vi "RampStateMachine.vi"(8 "error in (no error)":errorcluster) -> (0 "error out":errorcluster)   [LabVIEW 2013]
doc: "Use this template to build a VI to use as a subVI."
uses:
  RampProgramModel/RampProgramModel.lvclass
  RampState.ctl
  RampProgramModel/RampProgramModel.lvclass/RampProgramModel.ctl
  <vilib>/Utility/file.llb/Read From Spreadsheet File (DBL).vi
  <vilib>/Utility/file.llb/Write To Spreadsheet File (string).vi
panel:
  in  "Clear Table":bool
  in  "Repeat Program":u32=1 min=1 max=1000 step=1
  out "Current Repeat":u32=1 min=1 max=1000 step=1
  out "Repeat Program ind":u32=1 min=1 max=1000 step=1
  in  "SaveProgram":bool
  in  "LoadProgram":bool
  in  "PauseProgram":bool
  out "Time Elapsed":dbl
  out "Cooling rate (°C/min)":dbl
  out "SP (°C)":dbl
  in  "StopProgram":bool
  in  "RunProgram":bool
  in  "Current Temperature":dbl(slide) scale=-50.0..20.0 scale format="%.1g"
  out "Status":string
  in  "stop":bool
  in  "Add Entry":bool
  out "Ramp Program Table":string[][](table)
  # "Hardware Abstraction"
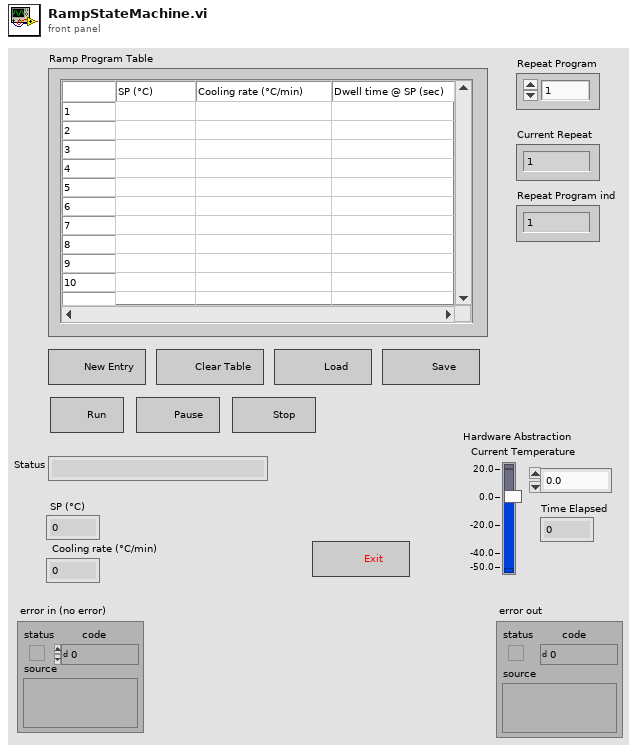
[diagram p1: front panel]
types:
  T1 = typedef "RampState.ctl" = enum16{"Pause Program", "Heatling/Cooling", "Dwelling @ SP", "Stopped"}
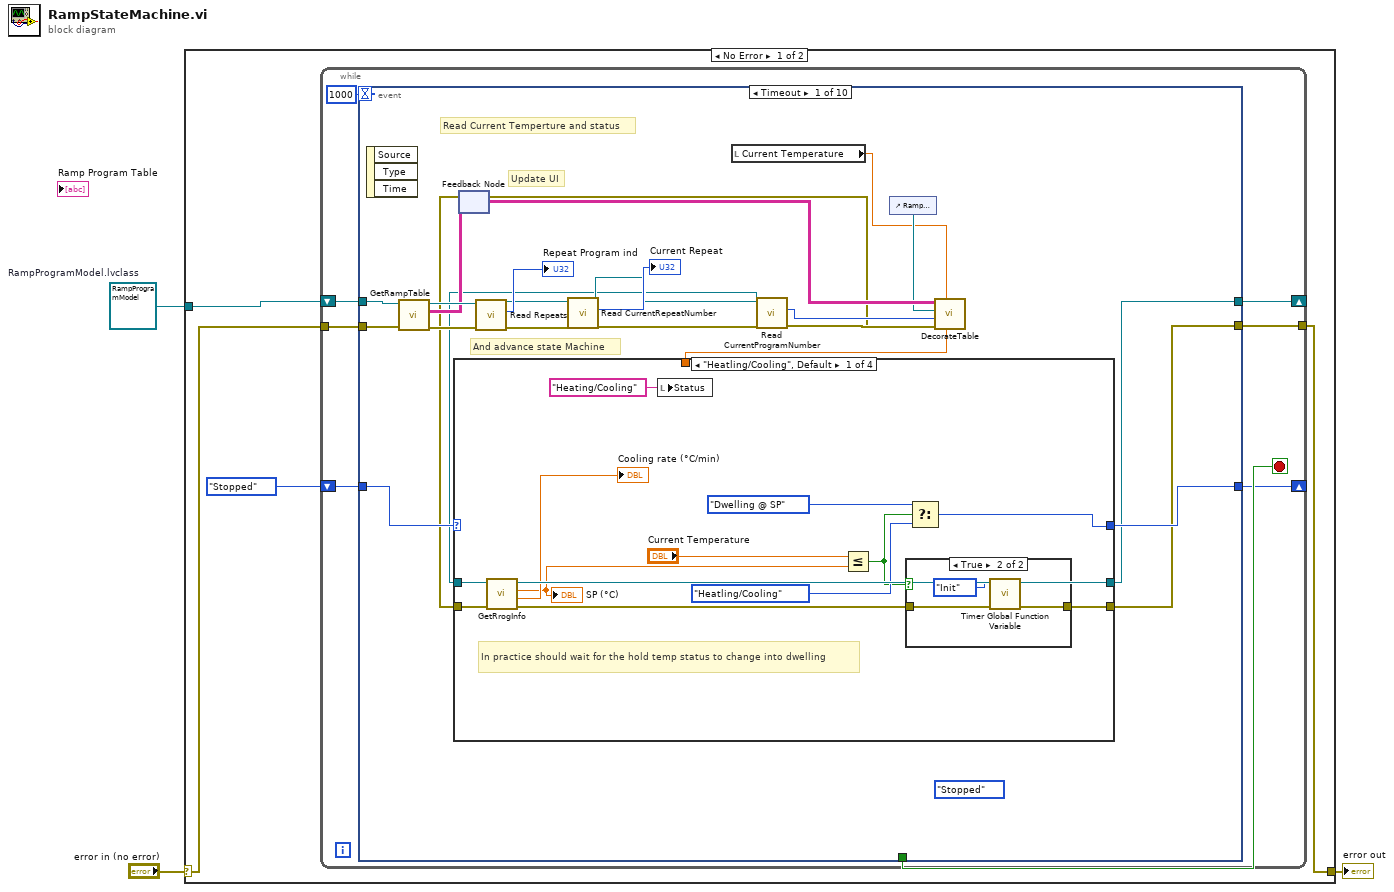
[diagram p0: block diagram]
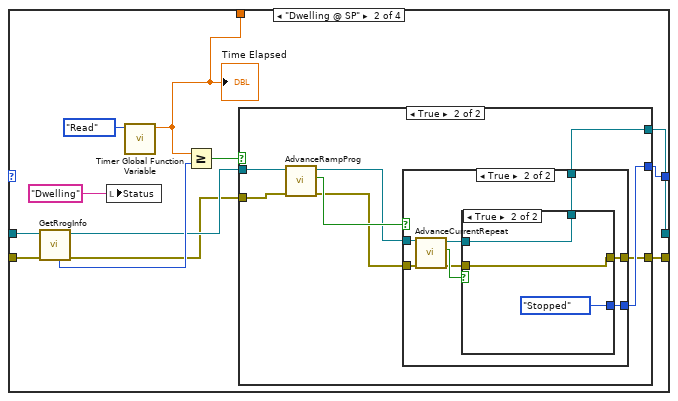
[diagram p3: hidden frame]
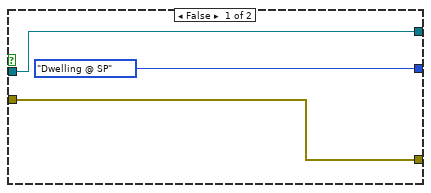
[diagram p4: hidden frame]
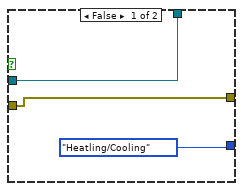
[diagram p5: hidden frame]
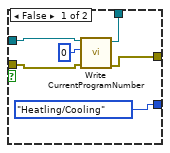
[diagram p6: hidden frame]
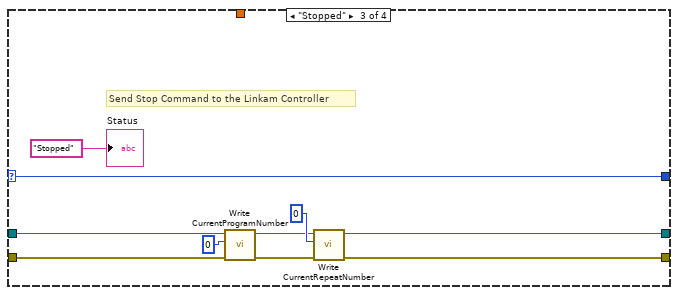
[diagram p7: hidden frame]
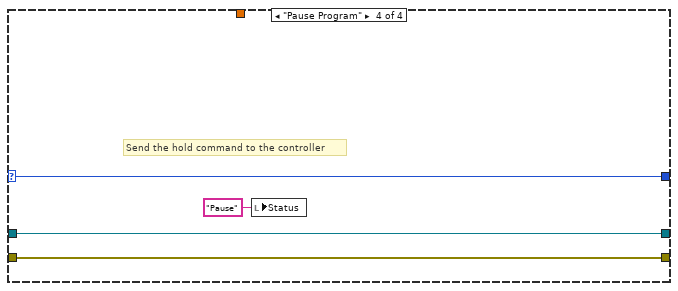
[diagram p8: hidden frame]
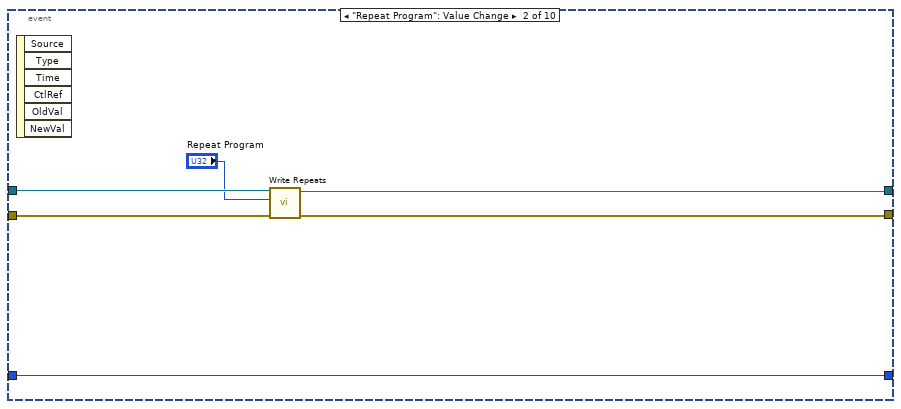
[diagram p9: hidden frame]
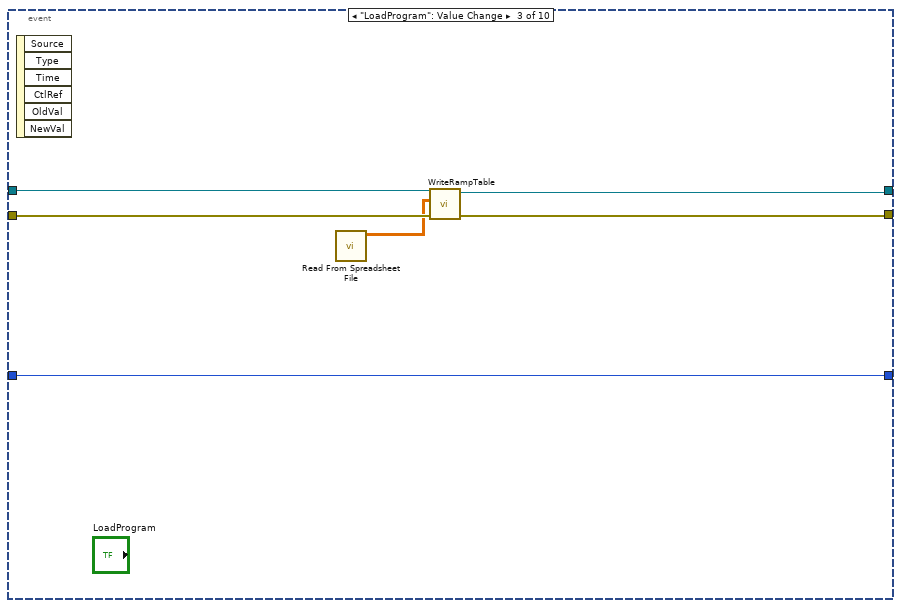
[diagram p10: hidden frame]
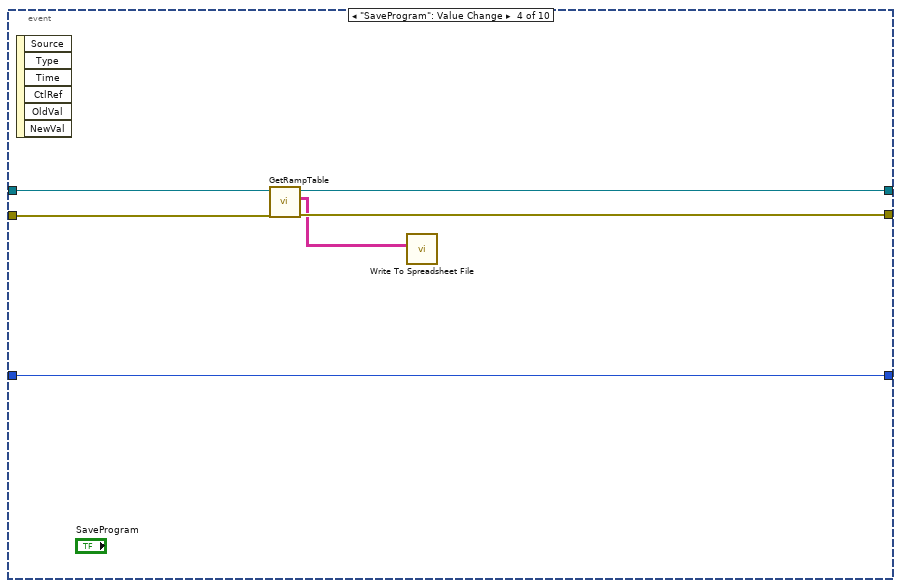
[diagram p11: hidden frame]
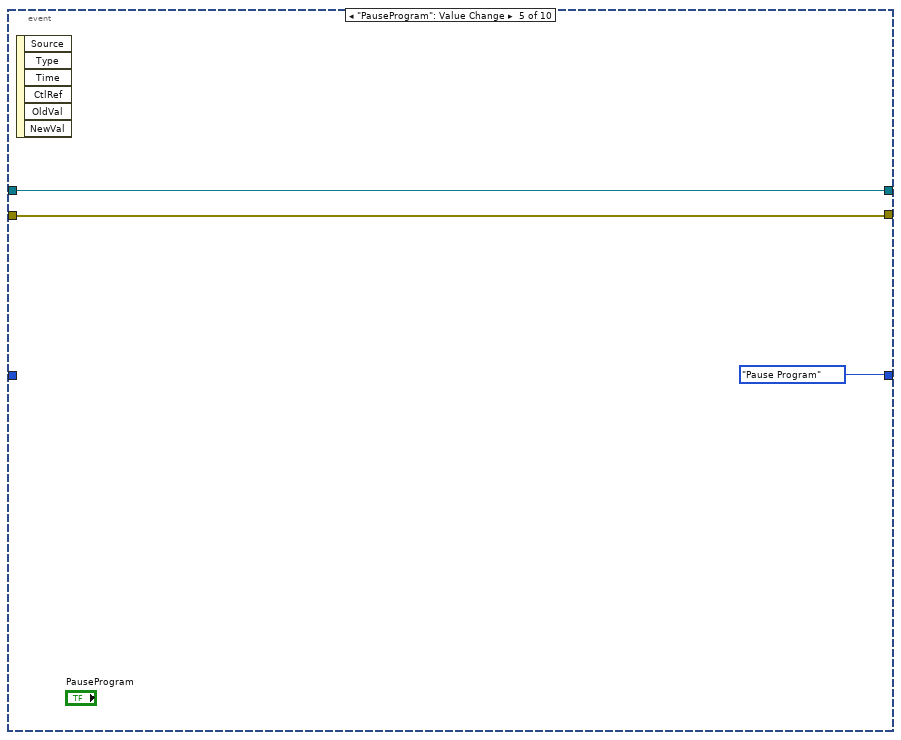
[diagram p12: hidden frame]
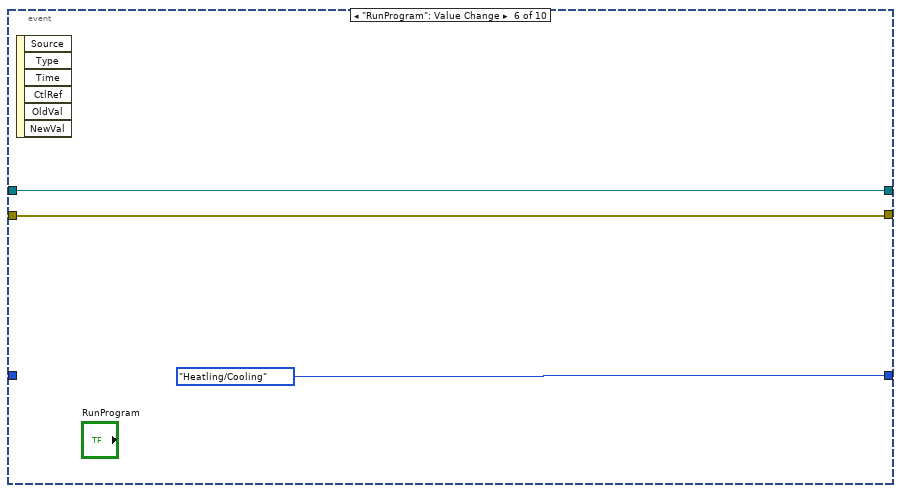
[diagram p13: hidden frame]
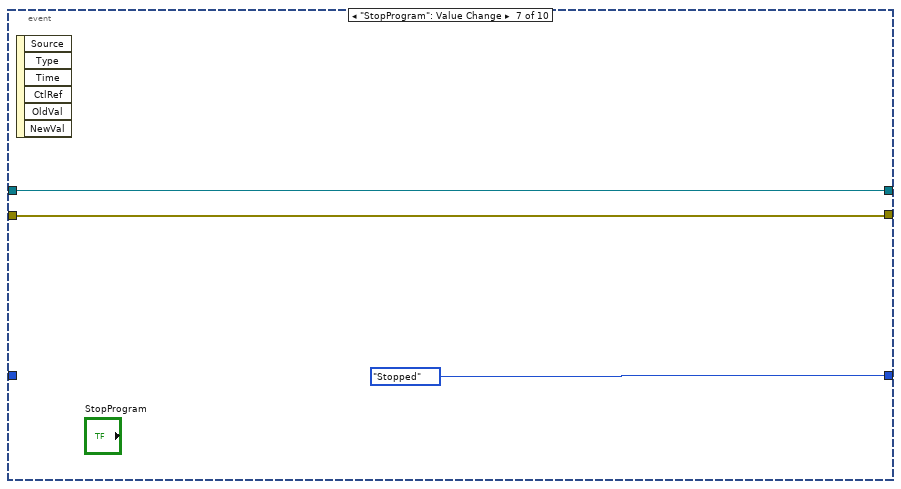
[diagram p14: hidden frame]
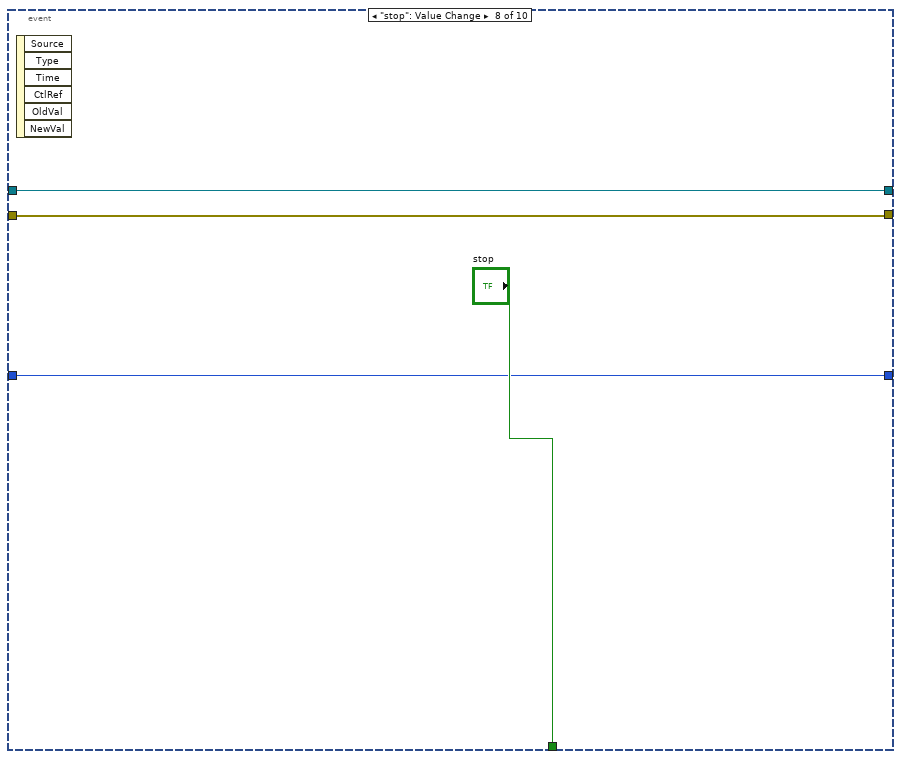
[diagram p15: hidden frame]
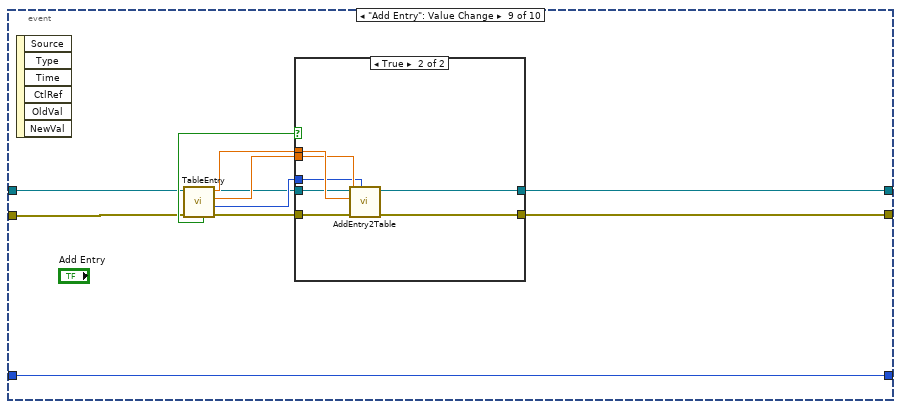
[diagram p16: hidden frame]
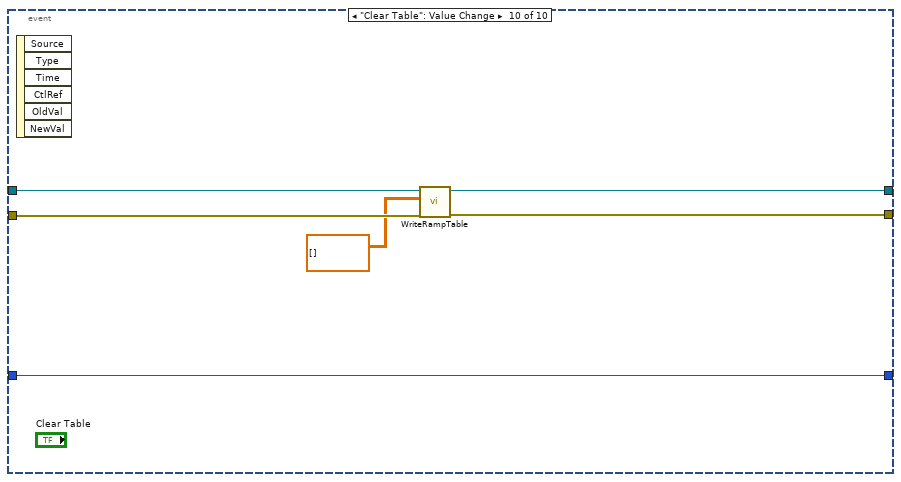
[diagram p18: hidden frame]
diagram:
  w1 = refnum<class "RampProgramModel.lvclass"> refnum  # RampProgramModel.lvclass
  n1 = case shown="No Error" "error in (no error)" {
    selector: "error in (no error)" -> [w7 w168]
    tunnel: [w6 w168] -> w2
    tunnel: w1 -> [w5 _]
    frame No Error {
      n2 = while {
        tunnel: w7 -> [w14]
        tunnel: [w13] -> w6
        shift-right: [w11] -> _
        shift-left: w5 -> [w12]
        shift-right: [w8] -> _
        shift-left: RampState."Stopped" ("State") -> [w9]
        stop <- w15 stop-if-true
        n3 = event shown="[0] Timeout" {
          selector: _ -> [_ _ _ _ _ _ _ _ _ _]
          dyn-events: _ -> [_ _ _ _ _ _ _ _ _ _]
          timeout: u32 1000 ("milliseconds to wait") -> [_ _ _ _ _ _ _ _ _ _]
          tunnel: [_ _ _ _ _ _ _ "stop" _ _] -> w15
          tunnel: w14 -> [w38 w117 w122 w127 w131 w133 w137 w141 w151 w165]
          tunnel: [w33 w116 w122 w125 w131 w133 w137 w141 w146 w164] -> w13
          tunnel: w12 -> [w37 w118 w121 w128 w132 w134 w136 w140 w144 w166]
          tunnel: [w34 w115 w120 w126 w132 w134 w136 w140 w145 w163] -> w11
          tunnel: w9 -> [w36 w113 w123 w129 _ _ _ w139 w143 w167]
          tunnel: [w35 w113 w123 w129 RampState."Pause Program" ("State") RampState."Heatling/Cooling" ("State") RampState."Stopped" ("State") w139 w143 w167] -> w8
          event Timeout {
            (unwired) RampState."Stopped" ("State")
            # "Read Current Temperture and status"
            # "And advance state Machine"
            # "Update UI"
            n4 = event-data() -> ()  [unwired: 1 in, 3 out]
            n5 = call "GetRampTable.vi"("error in (no error)"=w38, "RampProgramModel in"=w37) -> ("error out"=w30:errorcluster, "RampTable"=w26:string[][], "RampProgramModel out"=w32:refnum<class "RampProgramModel.lvclass">)  [unwired: 7 in]
            n6 = feedback #1() -> (w16:errorcluster)  [unwired: 1 in]
            n7 = call "Read Repeats.vi"("error in (no error)"=w30, "RampProgramModel in"=w32) -> ("error out"=w28:errorcluster, "Repeats"=→"Repeat Program ind":u32, "RampProgramModel out"=w29:refnum<class "RampProgramModel.lvclass">)  [unwired: 7 in]
            n8 = call "Read CurrentRepeatNumber.vi"("error in (no error)"=w28, "RampProgramModel in"=w29) -> ("error out"=w22:errorcluster, "CurrentRepeatNumber"=→"Current Repeat":u32, "RampProgramModel out"=w23:refnum<class "RampProgramModel.lvclass">)  [unwired: 7 in]
            n9 = local read "Current Temperature"() -> (w19:dbl)
            n10 = call "Read CurrentProgramNumber.vi"("error in (no error)"=w22, "RampProgramModel in"=w23) -> ("error out"=w18:errorcluster, "CurrentProgramNumber"=w20:u32, "RampProgramModel out"=w21:refnum<class "RampProgramModel.lvclass">)  [unwired: 7 in]
            n11 = case shown="\"Heatling/Cooling\", Default" w36 {
              selector: w36 -> [_ _ w108 w110]
              tunnel: [w44 w61 w108 w110] -> w35
              tunnel: w21 -> [w50 w66 w106 w109]
              tunnel: [w49 w58 w99 w109] -> w34
              tunnel: w16 -> [w48 w65 w104 w111]
              tunnel: [w39 w57 w100 w111] -> w33
              tunnel: [_ w56 _ _] -> w24
              frame "Heatling/Cooling", Default {
                # "In practice should wait for the hold temp status to change into dwelling"
                n12 = call "GetRrogInfo.vi"("error in (no error)"=w48, "RampProgramModel in"=w50) -> ("error out"=w40:errorcluster, "Cooling rate (°C/min)"=→"Cooling rate (°C/min)":dbl, "SP (°C)"=w42:dbl, "RampProgramModel out"=w49:refnum<class "RampProgramModel.lvclass">)  [unwired: 5 in, 1 out]
                "SP (°C)" <- w42
                n13 = local write "Status"("Heating/Cooling" ("Status")) -> ()
                n14 = Less Or Equal?(x="Current Temperature", y=w42) -> (x <= y?=w41:bool)
                n15 = case shown="True" w41 {
                  tunnel: w40 -> [w52 w54]
                  tunnel: [w52 w53] -> w39
                  frame False {
                  }
                  frame True {
                    n16 = call "Timer Global Function Variable.vi"("error in (no error)"=w54, "Enum"=enum16{"Init", "Read", "Set"}."Init") -> ("error out"=w53:errorcluster)  [unwired: 7 in, 2 out]
                  }
                }
                n17 = Select(t=RampState."Dwelling @ SP" ("State"), s=w41, f=RampState."Heatling/Cooling" ("State")) -> (s? t:f=w44:T1)
              }
              frame "Dwelling @ SP" {
                n18 = call "GetRrogInfo.vi"("error in (no error)"=w65, "RampProgramModel in"=w66) -> ("error out"=w59:errorcluster, "RampProgramModel out"=w60:refnum<class "RampProgramModel.lvclass">, "Dwell Time @ SP (sec)"=w63:u32)  [unwired: 5 in, 2 out]
                n19 = local write "Status"("Dwelling" ("Status")) -> ()
                n20 = call "Timer Global Function Variable.vi"("Enum"=enum16{"Init", "Read", "Set"}."Read") -> ("Time Elapsed"=w56:dbl)  [unwired: 8 in, 2 out]
                "Time Elapsed" <- w56
                n21 = Greater Or Equal?(x=w56, y=w63) -> (x >= y?=w62:bool)
                n22 = case shown="True" w62 {
                  tunnel: [RampState."Dwelling @ SP" ("State") w73] -> w61
                  tunnel: w60 -> [w69 w78]
                  tunnel: w59 -> [w68 w77]
                  tunnel: [w69 w72] -> w58
                  tunnel: [w68 w71] -> w57
                  frame False {
                  }
                  frame True {
                    n23 = call "AdvanceRampProg.vi"("error in (no error)"=w77, "RampProgramModel in"=w78) -> ("error out"=w74:errorcluster, "EndOfPrograms"=w76:bool, "RampProgramModel out"=w75:refnum<class "RampProgramModel.lvclass">)  [unwired: 7 in]
                    n24 = case shown="True" w76 {
                      tunnel: w75 -> [w79 w89]
                      tunnel: w74 -> [w80 w88]
                      tunnel: [RampState."Heatling/Cooling" ("State") w84] -> w73
                      tunnel: [w79 w83] -> w72
                      tunnel: [w80 w82] -> w71
                      frame False {
                      }
                      frame True {
                        n25 = call "AdvanceCurrentRepeat.vi"("error in (no error)"=w88, "RampProgramModel in"=w89) -> ("error out"=w85:errorcluster, "EndOfRepeats"=w87:bool, "RampProgramModel out"=w86:refnum<class "RampProgramModel.lvclass">)  [unwired: 7 in]
                        n26 = case shown="True" w87 {
                          tunnel: w86 -> [w93 w96]
                          tunnel: w85 -> [w92 w97]
                          tunnel: [RampState."Heatling/Cooling" ("State") RampState."Stopped" ("State")] -> w84
                          tunnel: [w90 w96] -> w83
                          tunnel: [w91 w97] -> w82
                          frame False {
                            n27 = call "Write CurrentProgramNumber.vi"("error in (no error)"=w92, "CurrentProgramNumber"=u32 0, "RampProgramModel in"=w93) -> ("error out"=w91:errorcluster, "RampProgramModel out"=w90:refnum<class "RampProgramModel.lvclass">)  [unwired: 7 in]
                          }
                          frame True {
                          }
                        }
                      }
                    }
                  }
                }
              }
              frame "Stopped" {
                # "Send Stop Command to the Linkam Controller"
                n28 = call "Write CurrentProgramNumber.vi"("error in (no error)"=w104, "CurrentProgramNumber"=u32 0, "RampProgramModel in"=w106) -> ("error out"=w101:errorcluster, "RampProgramModel out"=w102:refnum<class "RampProgramModel.lvclass">)  [unwired: 7 in]
                n29 = call "Write CurrentRepeatNumber.vi"("error in (no error)"=w101, "CurrentRepeatNumber"=u32 0, "RampProgramModel in"=w102) -> ("error out"=w100:errorcluster, "RampProgramModel out"=w99:refnum<class "RampProgramModel.lvclass">)  [unwired: 7 in]
                "Status" <- "Stopped" ("Status")
              }
              frame "Pause Program" {
                # "Send the hold command to the controller"
                n30 = local write "Status"("Pause" ("Status")) -> ()
              }
            }
            n31 = control-ref of="Ramp Program Table"() -> (w25:refnum<vi>)
            n32 = call "DecorateTable.vi"("Elapsed Time"=w24, "Current Temperature"=w19, "error in (no error)"=w18, "Current Program"=w20, "Tbl Refnum"=w25, "RampTable"=w26) -> ("error out"=w17:errorcluster)  [unwired: 5 in]
            n33 = feedback-in #1(w17) -> ()
          }
          event "Repeat Program": Value Change {
            n34 = event-data() -> ()  [unwired: 1 in, 6 out]
            n35 = call "Write Repeats.vi"("error in (no error)"=w117, "Repeats"="Repeat Program", "RampProgramModel in"=w118) -> ("error out"=w116:errorcluster, "RampProgramModel out"=w115:refnum<class "RampProgramModel.lvclass">)  [unwired: 7 in]
          }
          event "LoadProgram": Value Change {
            n36 = event-data() -> ()  [unwired: 1 in, 6 out]
            n37 = call-poly <vilib>:"Read From Spreadsheet File.vi"() -> ("all rows"=w119:dbl[][])  [unwired: 7 in, 4 out]
            n38 = call "WriteRampTable.vi"("RampFromFile"=w119, "RampProgramModel in"=w121) -> ("RampProgramModel out"=w120:refnum<class "RampProgramModel.lvclass">)  [unwired: 8 in, 1 out]
          }
          event "SaveProgram": Value Change {
            n39 = event-data() -> ()  [unwired: 1 in, 6 out]
            n40 = call "GetRampTable.vi"("error in (no error)"=w127, "RampProgramModel in"=w128) -> ("error out"=w125:errorcluster, "RampTable"=w124:string[][], "RampProgramModel out"=w126:refnum<class "RampProgramModel.lvclass">)  [unwired: 7 in]
            n41 = call-poly <vilib>:"Write To Spreadsheet File.vi"("2D data"=w124) -> ()  [unwired: 7 in, 1 out]
          }
          event "PauseProgram": Value Change {
            n42 = event-data() -> ()  [unwired: 1 in, 6 out]
          }
          event "RunProgram": Value Change {
            n43 = event-data() -> ()  [unwired: 1 in, 6 out]
          }
          event "StopProgram": Value Change {
            n44 = event-data() -> ()  [unwired: 1 in, 6 out]
          }
          event "stop": Value Change {
            n45 = event-data() -> ()  [unwired: 1 in, 6 out]
          }
          event "Add Entry": Value Change {
            n46 = event-data() -> ()  [unwired: 1 in, 6 out]
            n47 = call "TableEntry.vi"("error in (no error)"=w151) -> ("error out"=w147:errorcluster, "Dwell Time @ SP (sec) 2"=w148:u32, "Cooling rate (°C/min) 2"=w149:dbl, "SP (°C) 2"=w150:dbl, "Add Entry Pressed?"=w152:bool)  [unwired: 6 in]
            n48 = case shown="True" w152 {
              tunnel: w150 -> [_ w161]
              tunnel: w149 -> [_ w160]
              tunnel: w148 -> [_ w159]
              tunnel: w147 -> [w154 w158]
              tunnel: [w154 w155] -> w146
              tunnel: w144 -> [w153 w157]
              tunnel: [w153 w156] -> w145
              frame False {
              }
              frame True {
                n49 = call "AddEntry2Table.vi"("Dwell Time @ SP (sec)"=w159, "error in (no error)"=w158, "Cooling rate (°C/min)"=w160, "SP (°C)"=w161, "RampProgramModel in"=w157) -> ("error out"=w155:errorcluster, "RampProgramModel out"=w156:refnum<class "RampProgramModel.lvclass">)  [unwired: 5 in]
              }
            }
          }
          event "Clear Table": Value Change {
            n50 = event-data() -> ()  [unwired: 1 in, 6 out]
            n51 = call "WriteRampTable.vi"("error in (no error)"=w165, "RampFromFile"=dbl[][] [], "RampProgramModel in"=w166) -> ("error out"=w164:errorcluster, "RampProgramModel out"=w163:refnum<class "RampProgramModel.lvclass">)  [unwired: 7 in]
          }
        }
      }
    }
    frame Error {
    }
  }
  "error out" <- w2
